vi "Pump Start Detector (Conti).vi"(6 "Reset":bool, 9 "Consec Samples":i32, 11 "Crossing?":bool) -> (3 "Restarts":u32)   [LabVIEW 2019]
uses:
  <vilib>/Platform/TimedLoop/XDataNode/timing_clust.ctl
  <vilib>/Platform/TimedLoop/XDataNode/nitl_modes.ctl
  <vilib>/Platform/TimedLoop/XDataNode/wakeup.ctl
  <vilib>/Platform/TimedLoop/XDataNode/XDataNode.xnode
  <vilib>/Platform/TimedLoop/XDataNode/XDNodeRunTimeDep.lvlib
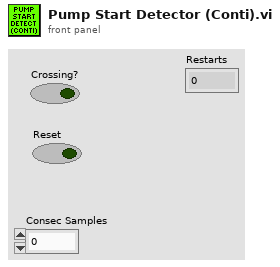
[diagram p1: front panel]
types:
  T1 = typedef "XDNodeRunTimeDep.lvlib/timing_clust.ctl" = cluster{"Expected End [f-1]":u64, "Actual End [f-1]":u64, "Finished Late? [f-1]":bool, "Expected End [i-1]":u64, "Actual End [i-1]":u64, "Finished Late? [i-1]":bool, "Expected Start [i]":u64, "Actual Start [i]":u64, "Expected Start [f]":u64, "Actual Start [f]":u64, "Source Name":string, "Structure Name":string, "Period":i64, "Deadline":i64, "Offset":i64, "Start":i64, "Priority":i32, "Timeout":i32, "Mode":T2, "Wakeup Reason":T3, "Error":errorcluster, "Source Type":string, "Secondary Source Type":string, "Global End Time":u64, "Global Start Time":u64, "Frame Duration":u64, "Iteration Duration":u64, "Assigned CPU":i32, "I/O Scan Engine Mode":u32}
  T2 = typedef "XDNodeRunTimeDep.lvlib/nitl_modes.ctl" = enum32{"No Change", "Process missed periods, maintain original phase", "Discard missed periods, maintain original phase", "Process missed periods, ignore original phase", "Discard missed periods, ignore original phase"}
  T3 = typedef "XDNodeRunTimeDep.lvlib/wakeup.ctl" = enum32{"Normal", "Aborted", "Asynchronous wakeup", "Timing source error", "Timed loop error", "Timeout"}
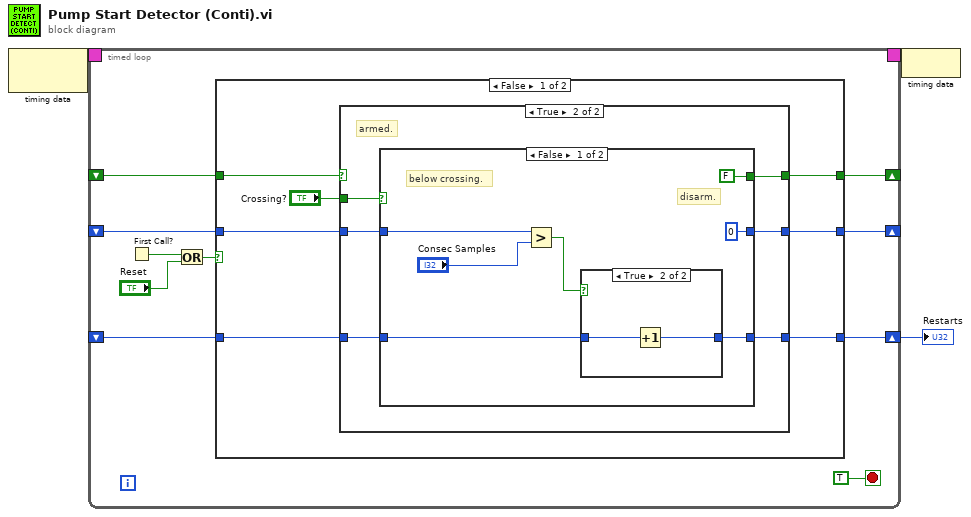
[diagram p0: block diagram]
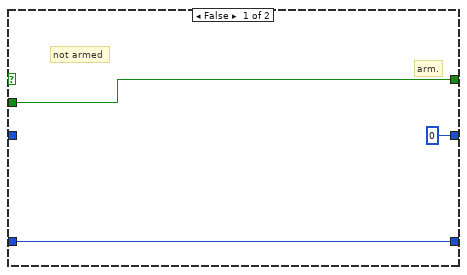
[diagram p2: hidden frame]
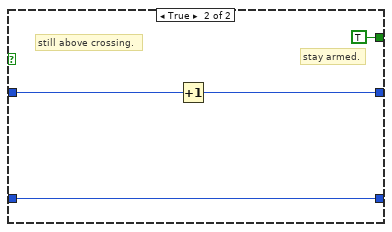
[diagram p4: hidden frame]
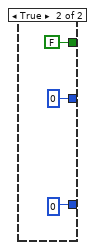
[diagram p5: hidden frame]
diagram:
  n1 = node-c288() -> (w3:T1)  [unwired: 1 in]
  n2 = timed-loop {
    shift-right: [w7] -> w1
    shift-left: _ -> [w8]
    shift-right: [w12] -> _
    shift-left: _ -> [w13]
    shift-right: [w11] -> _
    shift-left: _ -> [w10]
    timing: w3 -> [_]
    timing-out: [_] -> w2
    stop <- TRUE stop-if-true
    n3 = First Call?() -> (First Call?: T/F=w6:bool)
    n4 = Or(x=w6, y="Reset") -> (x .or. y?=w5:bool)
    n5 = case shown="False" w5 {
      tunnel: w13 -> [w20 _]
      tunnel: [w19 FALSE] -> w12
      tunnel: [w18 0] -> w11
      tunnel: w10 -> [w17 _]
      tunnel: w8 -> [w16 _]
      tunnel: [w15 u32 0] -> w7
      frame False {
        n6 = case shown="True" w20 {
          tunnel: [w23 w28] -> w19
          tunnel: [0 w27] -> w18
          tunnel: w17 -> [_ w26]
          tunnel: "Crossing?" -> [w23 w29]
          tunnel: w16 -> [w21 w25]
          tunnel: [w21 w24] -> w15
          frame False {
            # "arm."
            # "not armed"
          }
          frame True {
            # "armed."
            n7 = case shown="False" w29 {
              tunnel: [FALSE TRUE] -> w28
              tunnel: [0 w41] -> w27
              tunnel: w26 -> [w30 w42]
              tunnel: w25 -> [w32 w40]
              tunnel: [w31 w40] -> w24
              frame False {
                # "disarm."
                # "below crossing."
                n8 = Greater?(x=w30, y="Consec Samples") -> (0:w33:bool)
                n9 = case shown="True" w33 {
                  tunnel: w32 -> [w37 w39]
                  tunnel: [w37 w38] -> w31
                  frame False {
                  }
                  frame True {
                    n10 = Increment(x=w39) -> (x+1=w38:u32)
                  }
                }
              }
              frame True {
                # "stay armed."
                # "still above crossing."
                n11 = Increment(x=w42) -> (x+1=w41:i32)
              }
            }
          }
        }
      }
      frame True {
      }
    }
  }
  "Restarts" <- w1
  n12 = node-c288(w2) -> ()
